vi "Write Sender.vi"(10 "Sender":refnum<class "Sender.lvclass">, 11 "Destroy Msg in":refnum<class "Destroy Msg.lvclass">) -> (3 "Destroy Msg out":refnum<class "Destroy Msg.lvclass">)   [LabVIEW 2025, in "jettl.lvlib" / "Destroy Msg.lvlib" / "Destroy Msg.lvclass"]
uses:
  Destroy Msg.lvclass
  Destroy Msg.lvclass/Destroy Msg.ctl
  Sender/Sender/Sender.lvclass
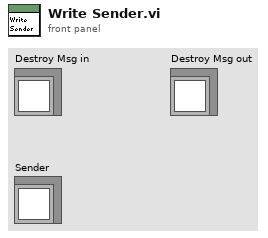
[diagram p1: front panel]
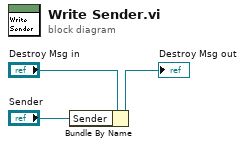
[diagram p0: block diagram]
diagram:
  n1 = Bundle By Name(cluster="Destroy Msg in", "Sender"="Sender") -> (→"Destroy Msg out":refnum<class "Destroy Msg.lvclass">)
